vi "Step Core.vi"(8 "error in (no error)":errorcluster, 11 "NULL_ADAPTER in":refnum<class "Null Adapter.lvclass">) -> (0 "error out":errorcluster, 3 "NULL_ADAPTER out":refnum<class "Null Adapter.lvclass">)   [LabVIEW 2018, in "Null Adapter.lvlib" / "Null Adapter.lvclass"]
uses:
  Null Adapter.lvclass
  Plugins/Measurement Interface.lvlibp/Measurement Interface.lvclass
  c:/Sequence Automation/Plugins/Measurement Interface.lvlibp/Measurement Interface.lvclass
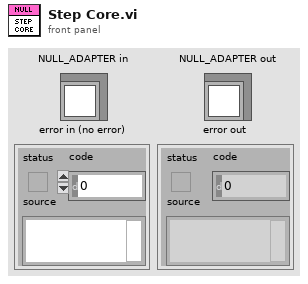
[diagram p1: front panel]
types:
  T1 = typedef "TestStand API Tools (TSAT).lvlibp/TSAT Evaluation Actions.lvlib/TSAT Evaluation.ctl" = cluster{"Test Name":string, "Pin":string, "Units":string, "SI Scaling":T2, "Test Number":i32, "Published Data Id":string, "Low Limit":dbl, "High Limit":dbl, "Export Data Location":string, "Software Bin":i64, "Evaluation Type":T3, "Test Data Source":string}
  T2 = typedef "TestStand API Tools (TSAT).lvlibp/TSAT Evaluation Actions.lvlib/TSAT Eval SI Unit Scaling.ctl" = i16
  T3 = typedef "TestStand API Tools (TSAT).lvlibp/TSAT Evaluation Actions.lvlib/TSAT Evaluation Type.ctl" = enum16{"Numeric Limit", "Pass/Fail", "None"}
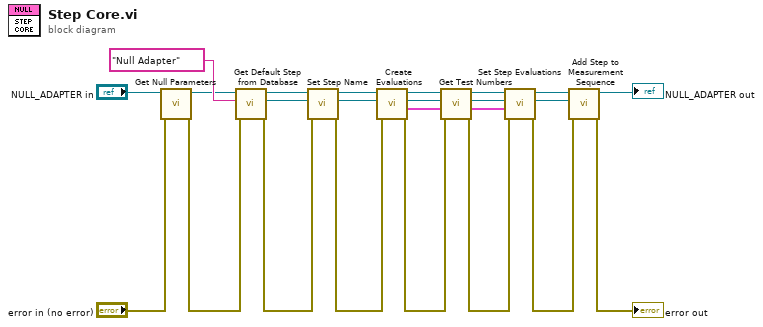
[diagram p0: block diagram]
diagram:
  n1 = call "Get Null Parameters.vi"("error in (no error)"="error in (no error)", "Null Adapter in"="NULL_ADAPTER in") -> ("error out"=w8:errorcluster, "Null Adapter out"=w2:refnum<class "Null Adapter.lvclass">)  [unwired: 8 in]
  n2 = call "Get Default Step from Database.vi"("error in (no error)"=w8, "Default Step"="Null Adapter", "Measurement Interface in"=w2) -> ("error out"=w4:errorcluster, "Cloned Step"=w6:refnum<k7>, "Measurement Interface out"=w1:refnum<class "Null Adapter.lvclass">)  [unwired: 6 in]
  n3 = call "Set Step Name.vi"("error in (no error)"=w4, "Step In"=w6, "NULL_ADAPTER in"=w1) -> ("error out"=w3:errorcluster, "Step Out"=w5:refnum<k7>, "NULL_ADAPTER out"=w7:refnum<class "Null Adapter.lvclass">)  [unwired: 6 in]
  n4 = call-dynamic "Create Evaluations.vi"("error in (no error)"=w3, "Null Adapter in"=w7) -> ("error out"=w16:errorcluster, "Evaluations Out"=w13:T1[], "Null Adapter out"=w17:refnum<class "Null Adapter.lvclass">)  [unwired: 7 in]
  n5 = call "Get Test Numbers.vi"("error in (no error)"=w16, "Evaluations In"=w13, "NULL_ADAPTER in"=w17) -> ("error out"=w14:errorcluster, "Evaluations Out"=w12:T1[], "NULL_ADAPTER out"=w15:refnum<class "Null Adapter.lvclass">)  [unwired: 6 in]
  n6 = call-dynamic "Set Step Evaluations.vi"("error in (no error)"=w14, "Evaluation Data"=w12, "Step In"=w5, "Null Adapter in"=w15) -> ("error out"=w19:errorcluster, "Step out"=w18:refnum<k7>, "Null Adapter out"=w20:refnum<class "Null Adapter.lvclass">)  [unwired: 5 in]
  n7 = call "Add Step to Measurement Sequence.vi"("error in (no error)"=w19, "Step to Add"=w18, "Measurement Interface in"=w20) -> ("error out"=→"error out":errorcluster, "Measurement Interface out"=→"NULL_ADAPTER out":refnum<class "Null Adapter.lvclass">)  [unwired: 7 in]
